vi "bmp085_get_cal_param.vi"(8 "error in (no error)":errorcluster, 11 "BMP085 (GY-65) in":refnum<class "BMP085 (GY-65).lvclass">) -> (0 "error out":errorcluster, 3 "BMP085 (GY-65) out":refnum<class "BMP085 (GY-65).lvclass">)   [LabVIEW 2015, in "BMP085 (RT).lvlib" / "BMP085 (GY-65).lvclass"]
uses:
  BMP085 (GY-65).lvclass
  BMP085 (GY-65).lvclass/BMP085 (GY-65).ctl
  <vilib>/Utility/error.llb/Error Cluster From Error Code.vi
  <vilib>/myRIO/Common/Instrument Driver Framework/myRIO v1.0/I2C/vis/myRIO v1.0 Write I2C.vi
  <vilib>/myRIO/Common/Instrument Driver Framework/myRIO v1.0/I2C/vis/myRIO v1.0 Read I2C.vi
  <vilib>/myRIO/Instrument Drivers/Onboard IO/I2C/I2C.lvlib
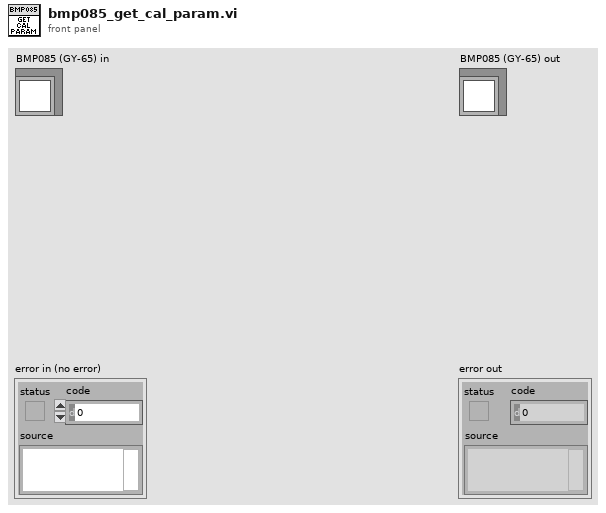
[diagram p1: front panel]
types:
  T1 = typedef "I2C.lvlib/I2C Reference.ctl" = cluster{"myRIO Reference":T2, "I2C Channels Enum":T6, "I2C Configuration":T7}
  T2 = typedef "myRIO Generic Hardware Reference.ctl" = cluster{"myRIO Model":T3, "myRIO Hardware Reference":T4}
  T3 = typedef "Hardware Version Enum.ctl" = enum16{"Unknown", "myRIO-1900", "myRIO-1950", "roboRIO"}
  T4 = typedef "myRIO v1.0 Reference.ctl" = cluster{"Generic FPGA Reference":T5, "Allow multiple opens":bool}
  T5 = typedef "Generic FPGA Reference.ctl" = refnum<k20>
  T6 = typedef "I2C Channels Enum.ctl" = enum16{"Not Connected", "A/I2C", "B/I2C", "I2C/I2C"}
  T7 = typedef "I2C.lvlib/I2C Configuration.ctl" = cluster{"I2C Transfer Rate":T8}
  T8 = typedef "I2C.lvlib/I2C Transfer Rate.ctl" = enum16{"Standard mode (100 kbps)", "Fast mode (400 kbps)"}
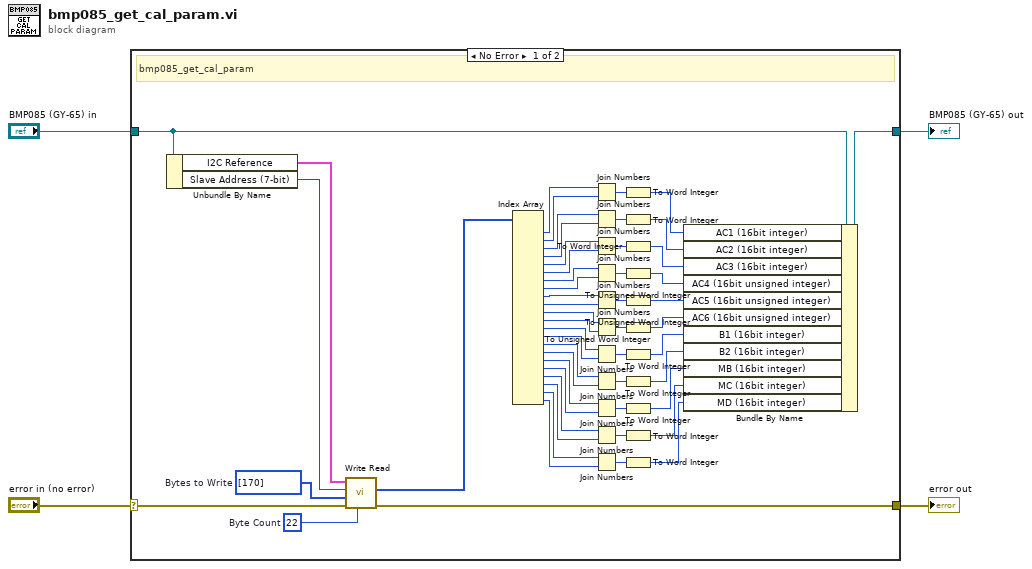
[diagram p0: block diagram]
diagram:
  n1 = case shown="No Error" "error in (no error)" {
    selector: "error in (no error)" -> [w53 w59]
    tunnel: [w52 w59] -> w3
    tunnel: [w50 w58] -> w1
    tunnel: "BMP085 (GY-65) in" -> [w55 w58]
    frame No Error {
      w56 = u8[] [170]  # Bytes to Write
      w57 = u32 22  # Byte Count
      # "bmp085_get_cal_param"
      n2 = Unbundle By Name(w55) -> ("I2C Reference"=w51:T1, "Slave Address (7-bit)"=w54:u8)
      n3 = call <vilib>:"Write Read.vi"("Byte Count"=w57, "error in (no error)"=w53, "Bytes to Write"=w56, "Slave Address (7-bit)"=w54, "I2C Ref In"=w51) -> ("error out"=w52:errorcluster, "Bytes Read"=w16:u8[])  [unwired: 3 in, 1 out]
      n4 = Index Array(array=w16) -> (element #1=w17:u8, element #2=w18:u8, element #3=w20:u8, element #4=w21:u8, element #5=w22:u8, element #6=w23:u8, element #7=w24:u8, element #8=w25:u8, element #9=w26:u8, element #10=w27:u8, element #11=w28:u8, element #12=w29:u8, element #13=w30:u8, element #14=w31:u8, element #15=w32:u8, element #16=w33:u8, element #17=w34:u8, element #18=w35:u8, element #19=w36:u8, element #20=w37:u8, element #21=w38:u8, element #22=w39:u8)  [unwired: 22 in]
      n5 = Join Numbers(hi=w17, lo=w18) -> ((hi.lo)=w19:u16)
      n6 = Join Numbers(hi=w20, lo=w21) -> ((hi.lo)=w40:u16)
      n7 = Join Numbers(hi=w22, lo=w23) -> ((hi.lo)=w41:u16)
      n8 = Join Numbers(hi=w24, lo=w25) -> ((hi.lo)=w42:u16)
      n9 = Join Numbers(hi=w26, lo=w27) -> ((hi.lo)=w43:u16)
      n10 = Join Numbers(hi=w28, lo=w29) -> ((hi.lo)=w44:u16)
      n11 = Join Numbers(hi=w30, lo=w31) -> ((hi.lo)=w45:u16)
      n12 = Join Numbers(hi=w32, lo=w33) -> ((hi.lo)=w46:u16)
      n13 = Join Numbers(hi=w34, lo=w35) -> ((hi.lo)=w47:u16)
      n14 = Join Numbers(hi=w36, lo=w37) -> ((hi.lo)=w48:u16)
      n15 = Join Numbers(hi=w38, lo=w39) -> ((hi.lo)=w49:u16)
      n16 = To Word Integer(number=w19) -> (16bit integer=w15:i16)
      n17 = To Word Integer(number=w40) -> (16bit integer=w14:i16)
      n18 = To Word Integer(number=w41) -> (16bit integer=w13:i16)
      n19 = To Unsigned Word Integer(number=w42) -> (unsigned 16bit integer=w12:u16)
      n20 = To Unsigned Word Integer(number=w43) -> (unsigned 16bit integer=w11:u16)
      n21 = To Unsigned Word Integer(number=w44) -> (unsigned 16bit integer=w10:u16)
      n22 = To Word Integer(number=w45) -> (16bit integer=w9:i16)
      n23 = To Word Integer(number=w46) -> (16bit integer=w8:i16)
      n24 = To Word Integer(number=w47) -> (16bit integer=w7:i16)
      n25 = To Word Integer(number=w48) -> (16bit integer=w6:i16)
      n26 = To Word Integer(number=w49) -> (16bit integer=w5:i16)
      n27 = Bundle By Name(cluster=w55, "AC1 (16bit integer)"=w15, "AC2 (16bit integer)"=w14, "AC3 (16bit integer)"=w13, "AC4 (16bit unsigned integer)"=w12, "AC5 (16bit unsigned integer)"=w11, "AC6 (16bit unsigned integer)"=w10, "B1 (16bit integer)"=w9, "B2 (16bit integer)"=w8, "MB (16bit integer)"=w7, "MC (16bit integer)"=w6, "MD (16bit integer)"=w5) -> (w50:refnum<class "BMP085 (GY-65).lvclass">)
    }
    frame Error {
    }
  }
  "error out" <- w3
  "BMP085 (GY-65) out" <- w1
